vi "InsertStrTo1DArrayCtrl.vi"(10 "문자열":string, 11 "array in":refnum<vi>) -> (3 "array out":refnum<vi>)   [LabVIEW 2018, in "Library-Ctrl.lvlib"]
uses:
  Library-Ctrl.lvlib
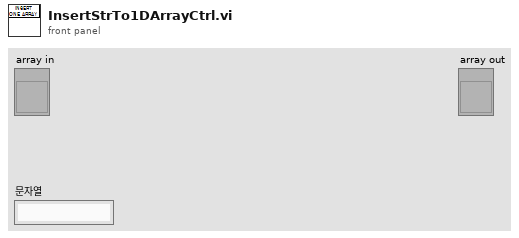
[diagram p1: front panel]
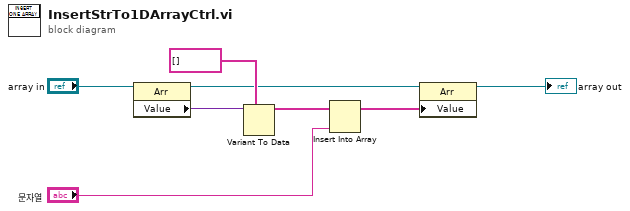
[diagram p0: block diagram]
diagram:
  n1 = property class="Arr"(reference="array in") -> (reference out=w3:refnum<vi>, "Value"=w7:variant)  [unwired: 1 in, 1 out]
  n2 = Variant To Data(type=string[] [], Variant=w7) -> (data=w5:string[])  [unwired: 1 in, 1 out]
  n3 = Insert Into Array(array=w5, new element="문자열") -> (w2:string[])  [unwired: 1 in]
  n4 = property class="Arr"(reference=w3, "Value"=w2) -> (reference out=→"array out":refnum<vi>)  [unwired: 1 in, 1 out]
